vi "Exit.vi"(8 "error in (no error)":errorcluster, 11 "Old State":refnum<class "Command Processor.lvclass">) -> (0 "error out":errorcluster, 3 "New State":refnum<class "Command Processor.lvclass">)   [LabVIEW 2013, in "Command Processor.lvlib" / "Command Processor.lvclass"]
doc: "This is an abstract method. Override this method to define the behavior when you leave the state."
uses:
  Command Processor.lvclass
  <vilib>/ni/Actors/State Actor/State Actor/State Actor.lvclass
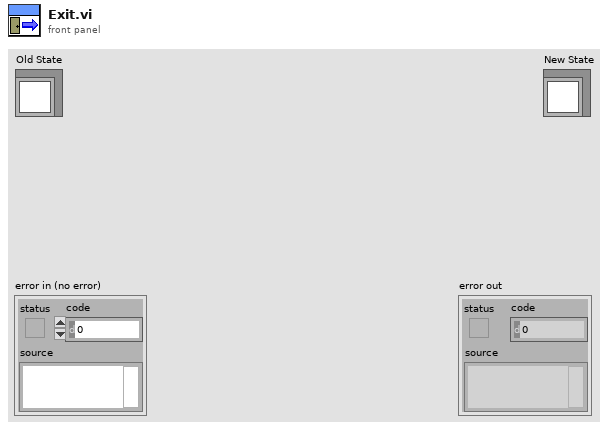
[diagram p1: front panel]
types:
  T1 = typedef "Command Processor.lvlib/Command Processor.lvclass/Command Processor Status.ctl" = cluster{"State Entry time":timestamp, "State Status":T2, "Command Processor Current State":string, "Command Status":T4}
  T2 = typedef "Current Previous State Status.ctl" = cluster{"Current State Status":T3, "Previous State Status":T3}
  T3 = typedef "State Status.ctl" = cluster{"State Name":string, "State Entry Time":timestamp, "State Exit Time":timestamp}
  T4 = typedef "Command Processor.lvlib/Command.lvlib/Command.lvclass/Command Status.ctl" = cluster{"Command Name":string, "Current State Status":T5, "Command Start Time":timestamp, "Command End Time":timestamp, "Previous State Status":T5}
  T5 = typedef "Command Processor.lvlib/Command.lvlib/Command.lvclass/State Status.ctl" = cluster{"State Name":string, "State Entry Time":timestamp, "State Exit Time":timestamp}
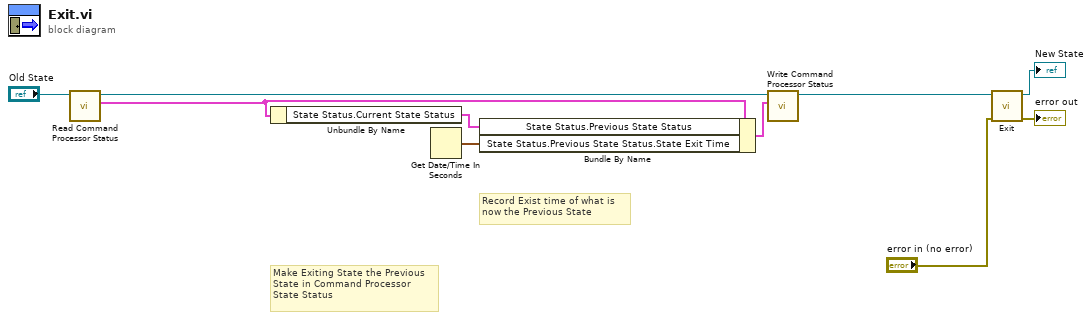
[diagram p0: block diagram]
diagram:
  # "Record Exist time of what is \nnow the Previous State"
  # "Make Exiting State the Previous\nState in Command Processor\nState Status"
  n1 = call-dynamic "Read Command Processor Status.vi"("Command Processor in"="Old State") -> ("Command Processor Status"=w4:T1, "Command Processor out"=w5:refnum<class "Command Processor.lvclass">)  [unwired: 8 in, 1 out]
  n2 = Unbundle By Name(w4) -> ("State Status.Current State Status"=w2:T3)
  n3 = Get Date/Time In Seconds() -> (seconds since 1Jan1904=w1:timestamp)
  n4 = Bundle By Name(cluster=w4, "State Status.Previous State Status"=w2, "State Status.Previous State Status.State Exit Time"=w1) -> (w3:T1)
  n5 = call-dynamic "Write Command Processor Status.vi"("Command Processor Status"=w3, "Command Processor in"=w5) -> ("Command Processor out"=w6:refnum<class "Command Processor.lvclass">)  [unwired: 8 in, 1 out]
  n6 = call-parent "Exit.vi"("error in (no error)"="error in (no error)", "Old State"=w6) -> ("error out"=→"error out":errorcluster, "New State"=→"New State":refnum<class "Command Processor.lvclass">)  [unwired: 8 in]
